vi "Collaborizm Temp Indicator Demo.vi"() -> ()   [LabVIEW 2014]
panel:
  in  "Stop Button":bool
  in  "Temp. Upper Limit":dbl
  out "Indicator":bool
  out "Thermometer":dbl(slide) scale=0.0..1000.0
  in  "Input Slider For Temp.":dbl(slide) scale=0.0..1000.0
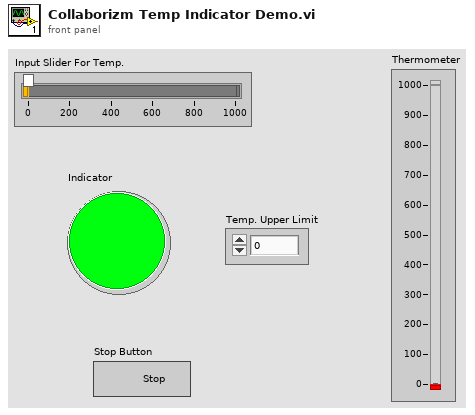
[diagram p1: front panel]
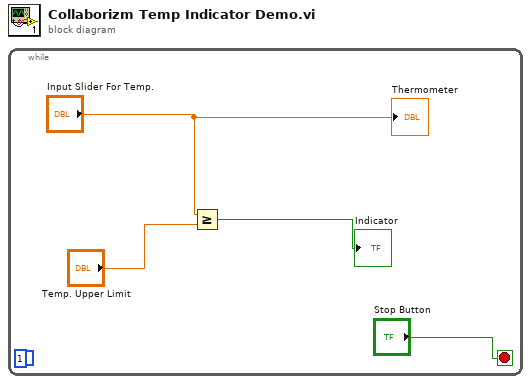
[diagram p0: block diagram]
diagram:
  n1 = while {
    stop <- "Stop Button" stop-if-true
    (unwired) 1
    n2 = Greater Or Equal?(x="Input Slider For Temp.", y="Temp. Upper Limit") -> (x >= y?=→"Indicator":bool)
    "Thermometer" <- "Input Slider For Temp."
  }
